vi "Recurse.vi"(0 "Combo index in":i32, 1 "Iterations array in":i32[](array[numeric]), 2 "Quantities":i32[](array[numeric]), 5 "Combos in":i32[][](array[numeric]), 7 "Values":i32[](array[numeric]), 9 "Goal amount":i32, 11 "Depth":i32, 12 "Result index in":i32, 13 "Results in":i32[][](array[numeric])) -> (4 "Progress - current iteration values":i32[](array[numeric]), 6 "Combo index out":i32, 8 "Combos out":i32[][](array[numeric]), 10 "Result index out":i32, 14 "Results out":i32[][](array[numeric]))   [LabVIEW 2018]
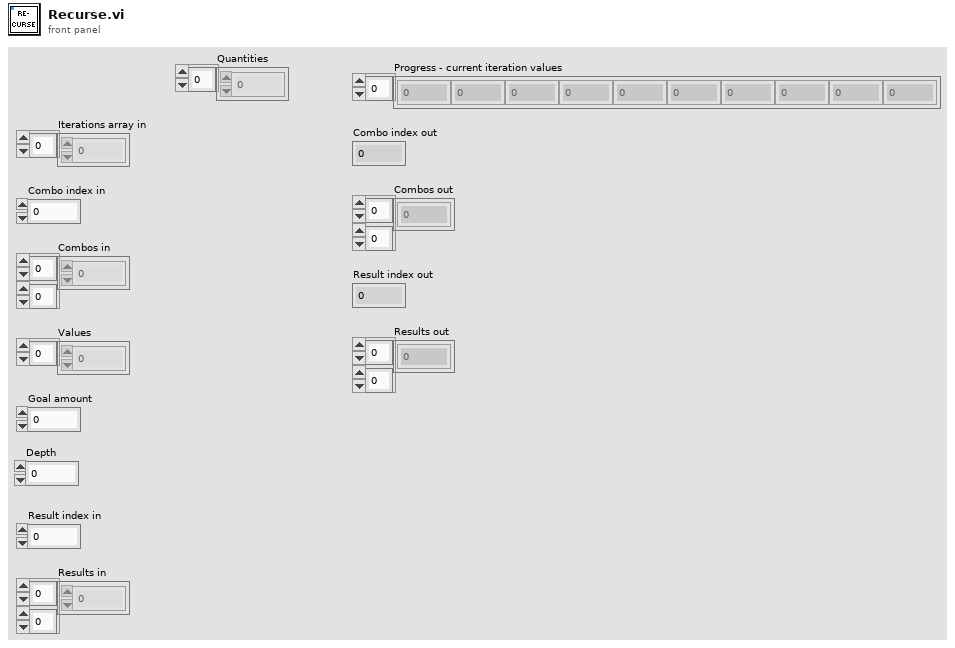
[diagram p1: front panel]
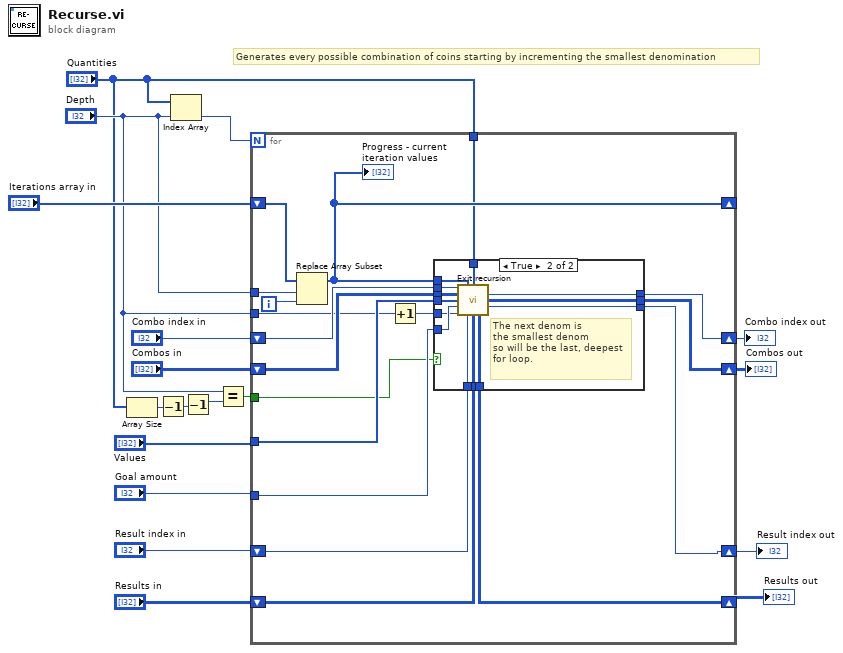
[diagram p0: block diagram]
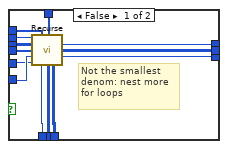
[diagram p2: hidden frame]
diagram:
  # "Generates every possible combination of coins starting by incrementing the smallest denomination"
  n1 = Array Size(array="Quantities") -> (size(s)=w3:i32)
  n2 = Decrement(x=w3) -> (x-1=w2:i32)
  n3 = Index Array(array="Quantities", index="Depth") -> (element=w7:i32)
  n4 = Decrement(x=w2) -> (x-1=w1:i32)
  n5 = Equal?(x="Depth", y=w1) -> (x = y?=w4:bool)
  n6 = for {
    N: w7 -> [_]
    shift-right: [w22] -> w8
    shift-left: "Combos in" -> [w36]
    shift-right: [w23] -> w11
    shift-left: "Combo index in" -> [w35]
    tunnel: "Values" -> [w28]
    shift-right: [w24] -> w16
    shift-left: "Result index in" -> [w25]
    shift-right: [w26] -> w15
    shift-left: "Results in" -> [w34]
    shift-right: [w30] -> _
    shift-left: "Iterations array in" -> [w31]
    tunnel: "Goal amount" -> [w27]
    tunnel: "Depth" -> [w32]
    tunnel: "Quantities" -> [w29]
    tunnel: "Depth" -> [w20]
    tunnel: w4 -> [w19]
    i -> [w33]
    n7 = Replace Array Subset(array=w31, new element=w33, index=w32) -> (w30:i32[])
    "Progress - current iteration values" <- w30
    n8 = Increment(x=w20) -> (x+1=w21:i32)
    n9 = case shown="True" w19 {
      tunnel: w36 -> [w46 w62]
      tunnel: w35 -> [w47 w61]
      tunnel: w34 -> [w44 w60]
      tunnel: w30 -> [w48 w59]
      tunnel: w29 -> [w49 w58]
      tunnel: w28 -> [w41 w57]
      tunnel: w27 -> [w40 w56]
      tunnel: [w43 w55] -> w26
      tunnel: w25 -> [w45 w54]
      tunnel: [w42 w53] -> w24
      tunnel: [w38 w52] -> w23
      tunnel: [w37 w51] -> w22
      tunnel: w21 -> [w39 w50]
      frame False {
        # "Not the smallest\ndenom: nest more\nfor loops"
        n10 = call "Recurse.vi"("Combo index in"=w47, "Iterations array in"=w48, "Quantities"=w49, "Combos in"=w46, "Values"=w41, "Goal amount"=w40, "Depth"=w39, "Result index in"=w45, "Results in"=w44) -> ("Combo index out"=w38:i32, "Combos out"=w37:i32[][], "Result index out"=w42:i32, "Results out"=w43:i32[][])  [unwired: 2 in, 1 out]
      }
      frame True {
        # "The next denom is\nthe smallest denom\nso will be the last, deepest\nfor loop."
        n11 = call "Exit recursion.vi"("combo index in"=w61, "Iterations array in"=w59, "Quantities"=w58, "Combos in"=w62, "Values"=w57, "Goal amount"=w56, "Depth"=w50, "Result index in"=w54, "Results in"=w60) -> ("Combo index out"=w52:i32, "Combos out"=w51:i32[][], "Result index out"=w53:i32, "Results out"=w55:i32[][])  [unwired: 2 in, 1 out]
      }
    }
  }
  "Result index out" <- w16
  "Results out" <- w15
  "Combo index out" <- w11
  "Combos out" <- w8
